vi "Rampa_Neg.vi"(0 "task/channels in":refnum<k21>, 1 "Start_A":dbl caption="Ángulo inicial" min=-5.0 max=5.0 step=0.05, 2 "Stop_A":dbl caption="Ángulo final" min=-5.0 max=5.0 step=0.05, 3 "Step_A":dbl=0.01 caption="Paso ángulo" min=0.01 max=1.0 step=0.05, 4 "ms to wait":u32=20 min=7 max=1000 step=1, 5 "Error In":errorcluster, 6 "# Ciclos":u16=1 min=1 max=20000 step=1) -> (19 "Error Out":errorcluster)   [LabVIEW 2016]
uses:
  Controles/Estados_RampaNEG.ctl
  <vilib>/DAQmx/write.llb/DAQmx Write (Analog DBL 1Chan 1Samp).vi
  <vilib>/DAQmx/miscellaneous.llb/DAQmx Fill In Error Info.vi
panel:
  out "OK":bool
  out "Volt":dbl caption="Voltaje (v)"
  in  "Cancel":bool
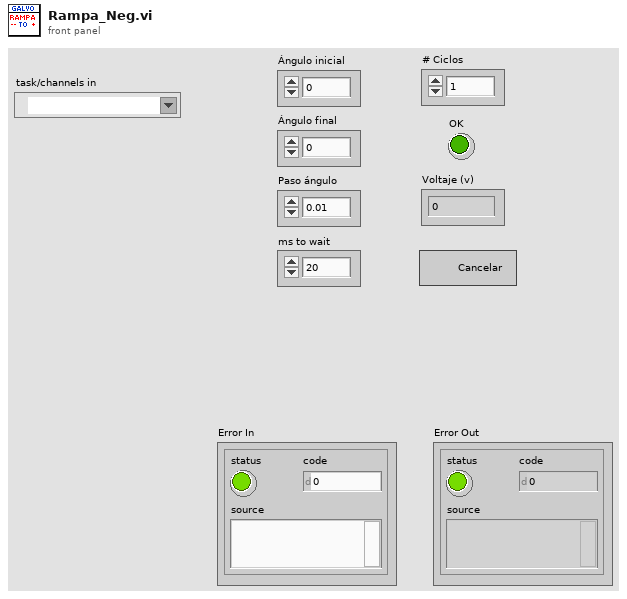
[diagram p1: front panel]
types:
  T1 = typedef "Estados_RampaNEG.ctl" = enum16{"Inicio", "Step+", "Ciclo+", "Step-", "Ciclo-"}
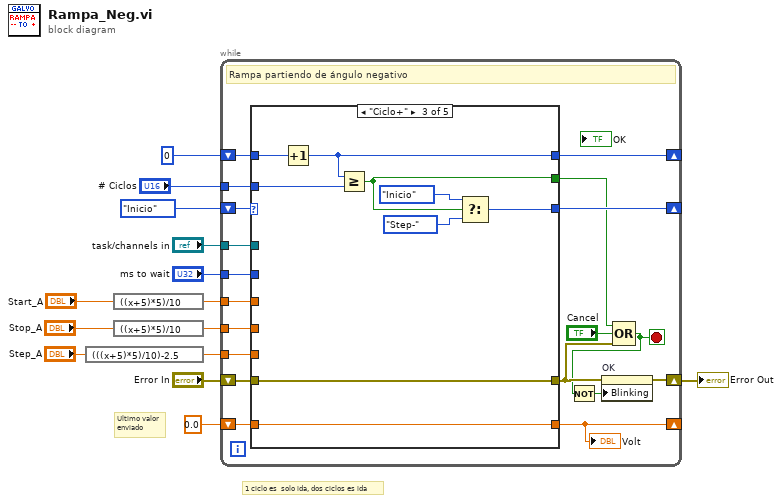
[diagram p0: block diagram]
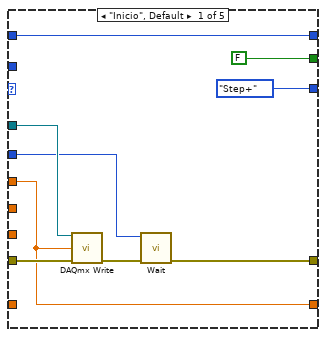
[diagram p2: hidden frame]
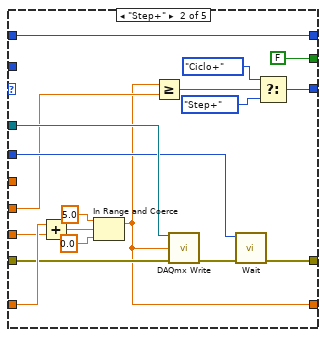
[diagram p3: hidden frame]
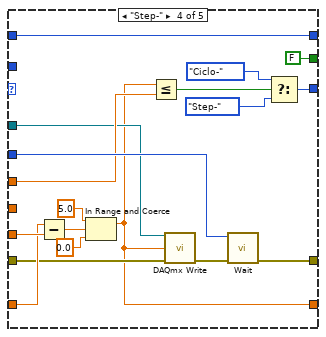
[diagram p4: hidden frame]
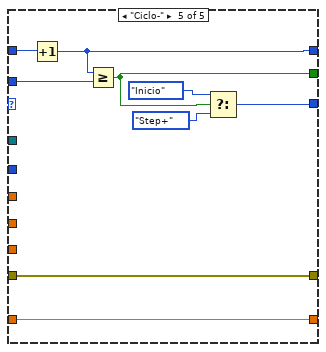
[diagram p5: hidden frame]
diagram:
  # "1 ciclo es  solo ida, dos ciclos es ida"
  # "Ultimo valor\nenviado"
  n1 = expression code="(((x+5)*5)/10)-2.5"("Step_A") -> (w9:dbl)
  n2 = expression code="((x+5)*5)/10"("Start_A") -> (w11:dbl)
  n3 = expression code="((x+5)*5)/10"("Stop_A") -> (w10:dbl)
  n4 = while {
    tunnel: w11 -> [w32]
    tunnel: w10 -> [w31]
    tunnel: w9 -> [w30]
    shift-right: [w26] -> _
    shift-left: Estados_RampaNEG."Inicio" -> [w33]
    shift-right: [w22] -> w3
    shift-left: "Error In" -> [w29]
    tunnel: "task/channels in" -> [w28]
    tunnel: "ms to wait" -> [w27]
    shift-right: [w23] -> _
    shift-left: 0.0 ("Start_A") -> [w25]
    tunnel: "# Ciclos" -> [w18]
    shift-right: [w16] -> _
    shift-left: u16 0 -> [w17]
    stop <- w19 stop-if-true
    # "Rampa partiendo de ángulo negativo"
    n5 = case shown="\"Ciclo+\"" w33 {
      tunnel: w32 -> [w37 _ _ w77 _]
      tunnel: w31 -> [_ w55 _ _ _]
      tunnel: w30 -> [_ w47 _ w87 _]
      tunnel: w29 -> [w42 w59 w67 w85 w88]
      tunnel: w28 -> [w41 w58 _ w76 _]
      tunnel: [w36 w50 w67 w78 w88] -> w21
      tunnel: w27 -> [w39 w56 _ w83 _]
      tunnel: [Estados_RampaNEG."Step+" w54 w63 w82 w95] -> w26
      tunnel: [w37 w45 w66 w72 w89] -> w23
      tunnel: w25 -> [_ w60 w66 w86 w89]
      tunnel: w18 -> [_ _ w68 _ w91]
      tunnel: w17 -> [w35 w44 w69 w70 w96]
      tunnel: [w35 w44 w61 w70 w90] -> w16
      tunnel: [FALSE FALSE w62 FALSE w92] -> w15
      frame "Inicio", Default {
        n6 = call-poly <vilib>:"DAQmx Write.vi"("task/channels in"=w41, "data"=w37, "error in"=w42) -> ("error out"=w40:errorcluster)  [unwired: 10 in, 2 out]
        n7 = call "Wait.vi"("Error In"=w40, "ms to wait"=w39) -> ("Error Out"=w36:errorcluster)  [unwired: 9 in]
      }
      frame "Step+" {
        n8 = Add(x=w60, y=w47) -> (x+y=w48:dbl)
        n9 = In Range and Coerce(upper limit=5.0, x=w48, lower limit=0.0) -> (coerced(x)=w45:dbl)  [unwired: 1 out]
        n10 = Greater Or Equal?(x=w45, y=w55) -> (x >= y?=w51:bool)
        n11 = call-poly <vilib>:"DAQmx Write.vi"("task/channels in"=w58, "data"=w45, "error in"=w59) -> ("error out"=w57:errorcluster)  [unwired: 10 in, 2 out]
        n12 = call "Wait.vi"("Error In"=w57, "ms to wait"=w56) -> ("Error Out"=w50:errorcluster)  [unwired: 9 in]
        n13 = Select(t=Estados_RampaNEG."Ciclo+", s=w51, f=Estados_RampaNEG."Step+") -> (s? t:f=w54:T1)
      }
      frame "Ciclo+" {
        n14 = Increment(x=w69) -> (x+1=w61:u16)
        n15 = Greater Or Equal?(x=w61, y=w68) -> (x >= y?=w62:bool)
        n16 = Select(t=Estados_RampaNEG."Inicio", s=w62, f=Estados_RampaNEG."Step-") -> (s? t:f=w63:T1)
      }
      frame "Step-" {
        n17 = Subtract(x=w86, y=w87) -> (x-y=w73:dbl)
        n18 = In Range and Coerce(upper limit=5.0, x=w73, lower limit=0.0) -> (coerced(x)=w72:dbl)  [unwired: 1 out]
        n19 = Less Or Equal?(x=w72, y=w77) -> (x <= y?=w79:bool)
        n20 = call-poly <vilib>:"DAQmx Write.vi"("task/channels in"=w76, "data"=w72, "error in"=w85) -> ("error out"=w84:errorcluster)  [unwired: 10 in, 2 out]
        n21 = call "Wait.vi"("Error In"=w84, "ms to wait"=w83) -> ("Error Out"=w78:errorcluster)  [unwired: 9 in]
        n22 = Select(t=Estados_RampaNEG."Ciclo-", s=w79, f=Estados_RampaNEG."Step-") -> (s? t:f=w82:T1)
      }
      frame "Ciclo-" {
        n23 = Increment(x=w96) -> (x+1=w90:u16)
        n24 = Greater Or Equal?(x=w90, y=w91) -> (x >= y?=w92:bool)
        n25 = Select(t=Estados_RampaNEG."Inicio", s=w92, f=Estados_RampaNEG."Step+") -> (s? t:f=w95:T1)
      }
    }
    "Volt" <- w23
    n26 = Compound Arithmetic op=OR(w15, "Cancel", w21) -> (w19:bool)
    n27 = Not(x=w19) -> (.not. x?=w20:bool)
    n28 = property on="OK" class="Bool (strict)"(error in=w21, "Blinking"=w20) -> (error out=w22:errorcluster)  [unwired: 1 in, 1 out]
  }
  "Error Out" <- w3
